vi "Simulated Car Client.vi"(7 "stop signal":refnum<user-event>, 10 "project namespace":string="LabVIEWDemo", 11 "Client Name":string="Car") -> ()   [LabVIEW 2017]
uses:
  Car/Car State -- enum.ctl
  TrafficMap/TrafficMap.lvclass/TrafficMap.ctl
  <vilib>/LabVIEW Open Source Project/MQTT Broker/Client/Client.lvclass
  C:/Program Files (x86)/National Instruments/LabVIEW 2017/vi.lib/LabVIEW Open Source Project/MQTT Broker/MQTT_Base/MQTT_Base.lvclass
  <vilib>/LabVIEW Open Source Project/MQTT Broker/Control Packets/PUBLISH/PUBLISH.lvclass
  C:/Program Files (x86)/National Instruments/LabVIEW 2017/vi.lib/LabVIEW Open Source Project/MQTT Broker/Control Packets/ControlPacket/ControlPacket.lvclass
  typedefs/Node Type -- enum.ctl
  TrafficMap/TrafficMap.lvclass
  typedefs/RequestPayload -- cluster.ctl
  typedefs/ResponsePayload -- cluster.ctl
  Serializer.JKI-JSON/Serializer.JKI-JSON.lvclass
  C:/Program Files (x86)/National Instruments/LabVIEW 2017/vi.lib/LabVIEW Open Source Project/Serializer/Serializer/Serializer.lvclass
  <vilib>/LabVIEW Open Source Project/MQTT Broker/MQTT_Base/MQTT_Base.lvclass/MQTT_Base.ctl
  <vilib>/LabVIEW Open Source Project/MQTT Broker/Client/Client.lvclass/Client.ctl
  <vilib>/LabVIEW Open Source Project/MQTT Broker/Control Packets/CONNECT/ConnectFlags -- cluster.ctl
  typedefs/ConnectPayload-- cluster.ctl
  typedefs/DisconnectPayload-- cluster.ctl
  <vilib>/LabVIEW Open Source Project/MQTT Broker/Control Packets/ControlPacket/ControlPacket.lvclass/ControlPacket.ctl
  0d705227-134d-4031-8d1e-e35da49b8ba8.vi
  580889ff-0a4c-41a4-b259-1db762517910.vi
  3d3687d4-2784-4a3f-94ff-e25152285f29.vi
  45bbbbd6-bbd6-4c9d-8aa1-54a553140d59.vi
  c7907ea9-6b4e-410e-be68-a96135e16753.vi
  a8e81dbf-d079-406f-abbd-3f6e0d275bc5.vi
  b830538a-2e83-4cc7-9605-dce1a29f0d38.vi
  <vilib>/LabVIEW Open Source Project/Serializer/Serializer.FlattenedString/Serializer.FlattenedString.lvclass
  <vilib>/LabVIEW Open Source Project/MQTT Broker/MQTT_Base/Decode Publish Package.vi
  <vilib>/LabVIEW Open Source Project/Serializer/Serializer/Serializer.lvclass
  <vilib>/LabVIEW Open Source Project/MQTT Broker/MQTT_Base/MQTT_Base.lvclass
  <vilib>/LabVIEW Open Source Project/MQTT Broker/Control Packets/ControlPacket/ControlPacket.lvclass
  <vilib>/LabVIEW Open Source Project/MQTT Broker/Control Packets/CONNECT/CONNECT.lvclass
  <vilib>/addons/_JKI.lib/Serialization/JSON/JKI JSON Serialization.lvlib
  Car/Car.lvclass
panel:
  out "Incoming topic":string
  out "Nb Cars in Current Zone":u32(knob) scale=0.0..10.0
  out "Zone registered":string
  in  "Map Update":bool
  out "Map":u16[][](graph)
  in  "Zones":u16(ring) items=["A", "B", "C", "D"]
  in  "Set Zone":bool
  in  "car state":T1
  in  "List Zones":bool
  out "Raw Packet String":string
  out "Payload":variant
  in  "Car Client Status":i32(listbox)
  out "Topic":string
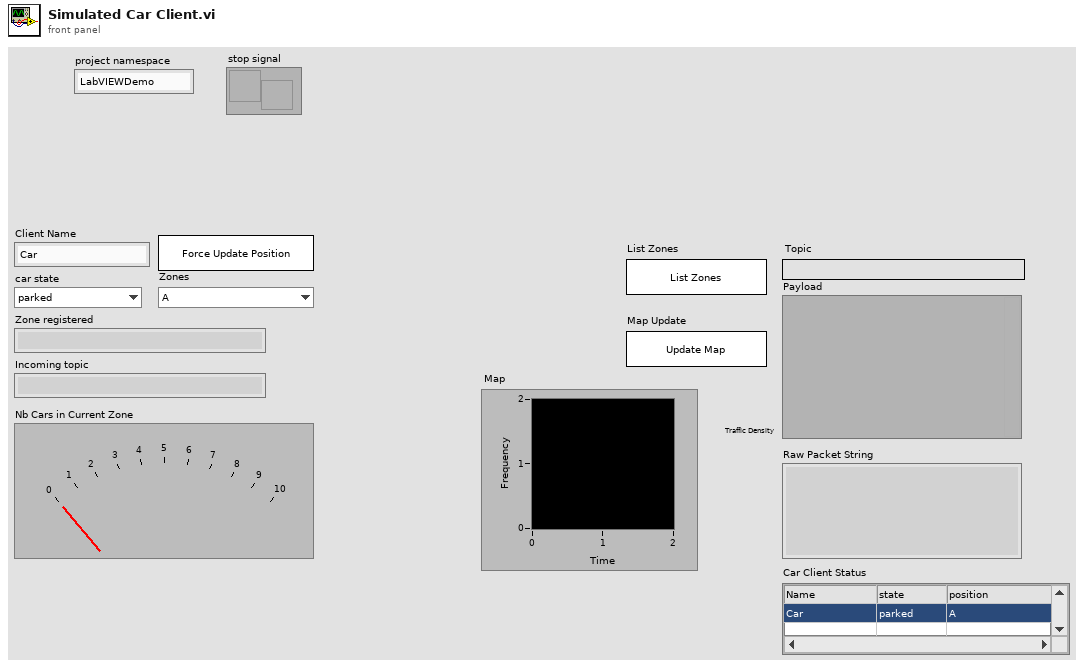
[diagram p1: front panel]
types:
  T1 = typedef "Car.lvclass/Car State -- enum.ctl" = enum16{"parked", "driving"}
  T2 = enum32{"Invalid", "Standard", "Closed", "Hidden", "Minimized", "Maximized"}
  T3 = enum32{"invalid app kind", "Development System", "Run Time System", "Student Edition", "Embedded LabVIEW", "Evaluation", "Custom"}
  T4 = typedef "ResponsePayload -- cluster.ctl" = cluster{"request":string, "reply":variant}
  T5 = typedef "CONNECT.lvclass/ConnectFlags -- cluster.ctl" = cluster{"Reserved":bool, "Clean Session":bool, "Will Flag":bool, "Will QoS 1":bool, "Will QoS 2":bool, "Will Retain":bool, "Password Flag":bool, "User Name Flag":bool}
  T6 = cluster{"Will Topic":string, "Will Message":string, "Username":string, "Password":string}
  T7 = typedef "RequestPayload -- cluster.ctl" = cluster{"request":string, "reply-to":string}
  T8 = typedef "ConnectPayload-- cluster.ctl" = cluster{"Node type":string}
  T9 = typedef "DisconnectPayload-- cluster.ctl" = cluster{"timestamp":string}
  T10 = typedef "Node Type -- enum.ctl" = enum16{"Car", "Hub", "Sensor", "Relay"}
  T11 = cluster{"Core":cluster{"Current VI Reference":refnum<vi>, "Close Panel on Exit?":bool}, "server address":string, "project namespace":string, "Client Name":string, "Node type":T10, "Client":refnum<class "Client.lvclass">, "Close on MQTT Disconnection?":bool, "Hub Name":string, "AppMessage":refnum<class "PUBLISH.lvclass">, "stop signal":refnum<user-event>, "TrafficMap":refnum<class "TrafficMap.lvclass">, "Request":T7}
  T12 = typedef "CONNACK.lvclass/Connect Return Code -- enum.ctl" = enum16{"Connection accepted", "Unacceptable protocol version", "Identifier Rejected", "Server Unavailable", "Bad Username or Password", "Not Authorized"}
  T13 = cluster{"Current VI Reference":refnum<vi>, "Close Panel on Exit?":bool}
  T14 = typedef "MQTT Server.lvlib/Client.lvclass/Public Events -- cluster.ctl" = cluster{"Connection Status":refnum<user-event>, "Connected":refnum<user-event>, "Application Message":refnum<user-event>}
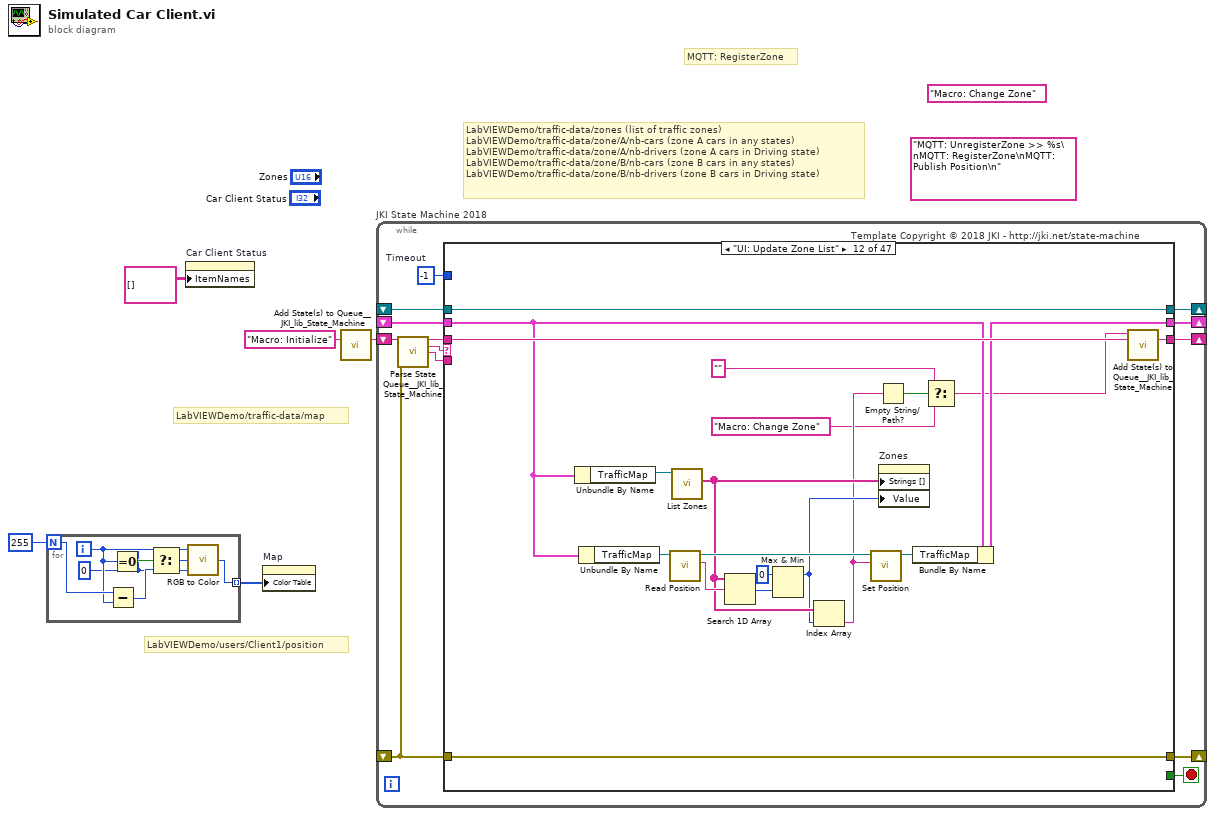
[diagram p0: block diagram]
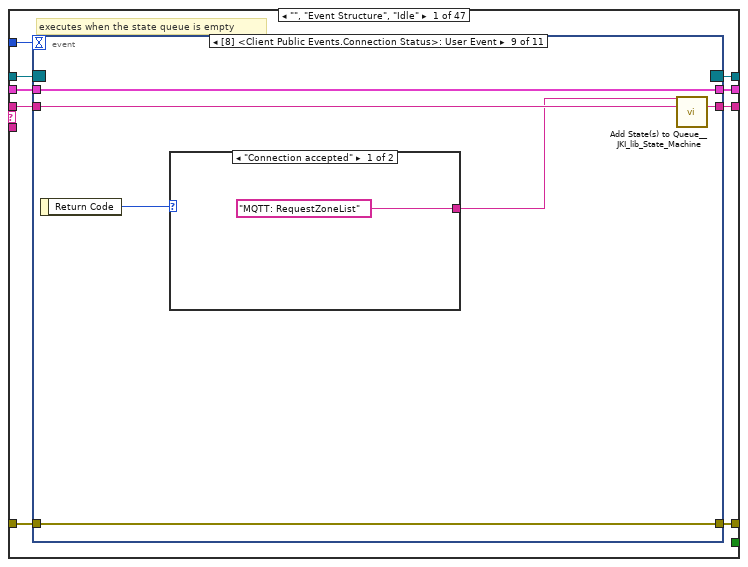
[diagram p2: hidden frame]
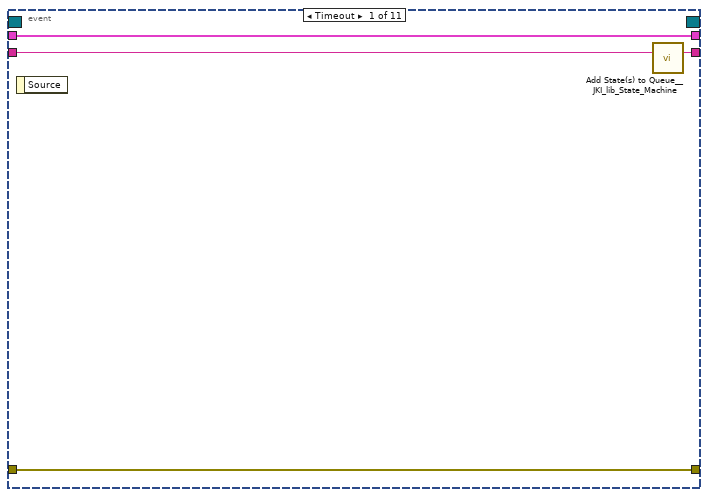
[diagram p3: hidden frame]
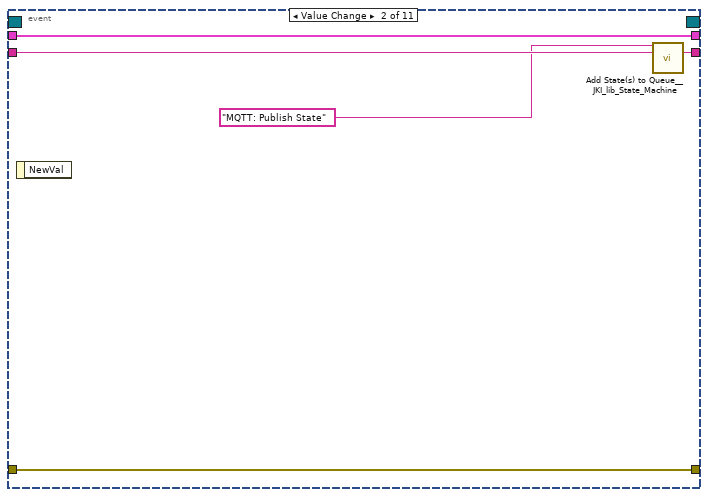
[diagram p4: hidden frame]
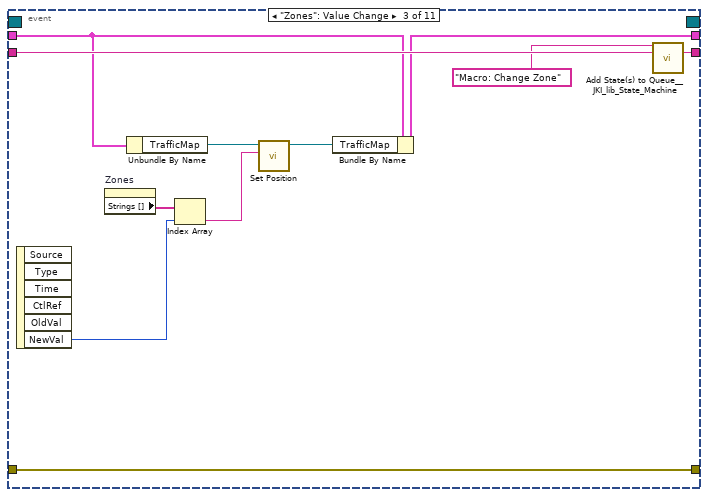
[diagram p5: hidden frame]
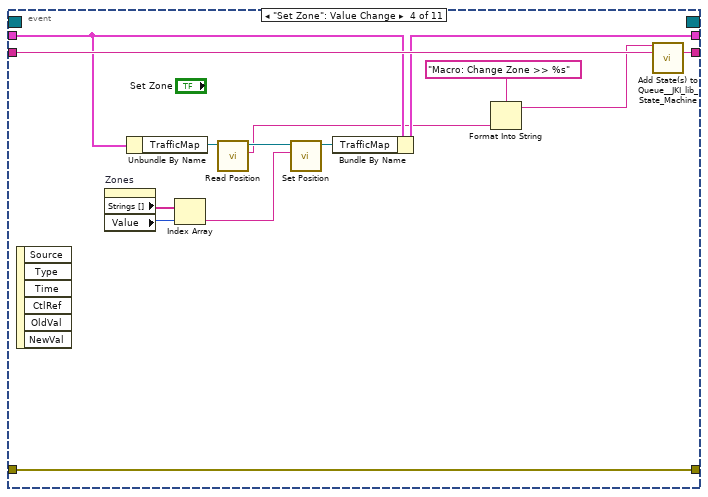
[diagram p6: hidden frame]
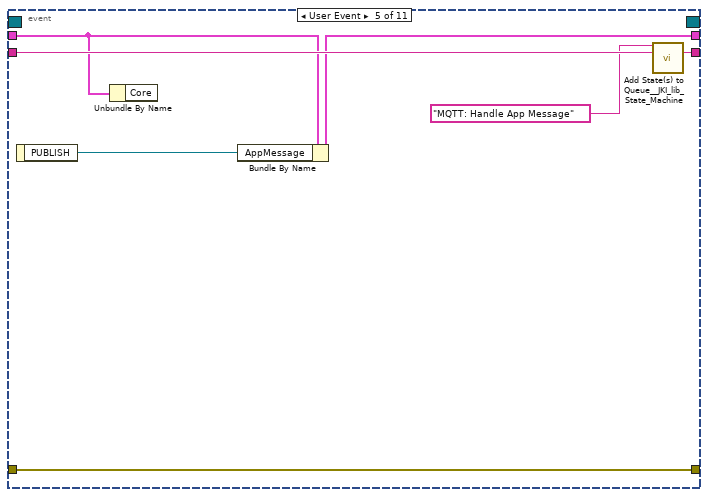
[diagram p7: hidden frame]
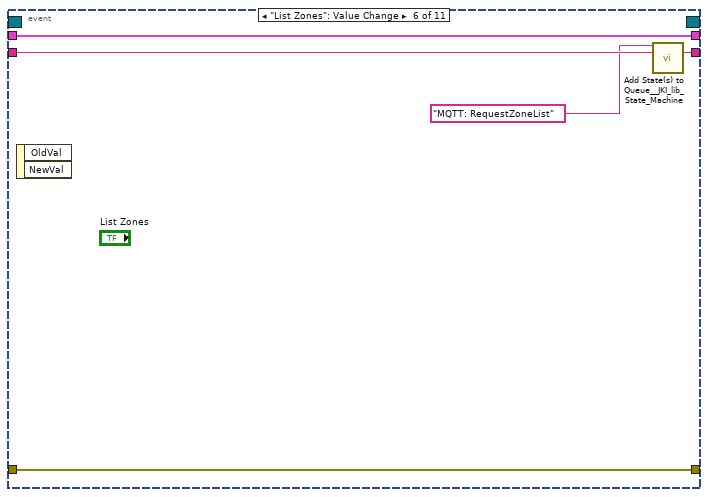
[diagram p8: hidden frame]
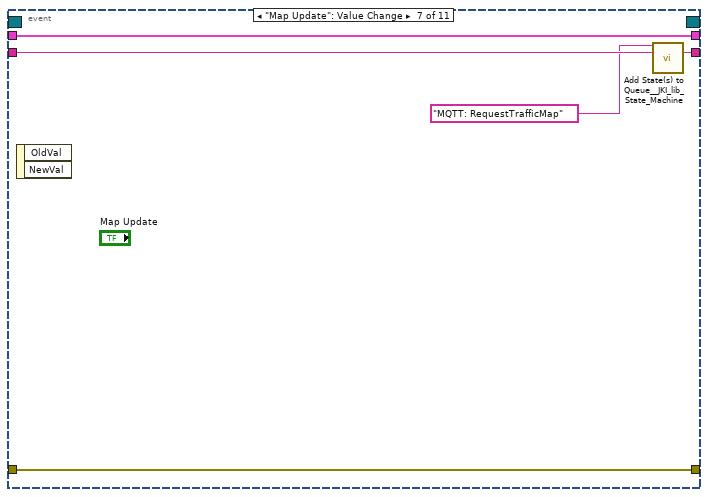
[diagram p9: hidden frame]
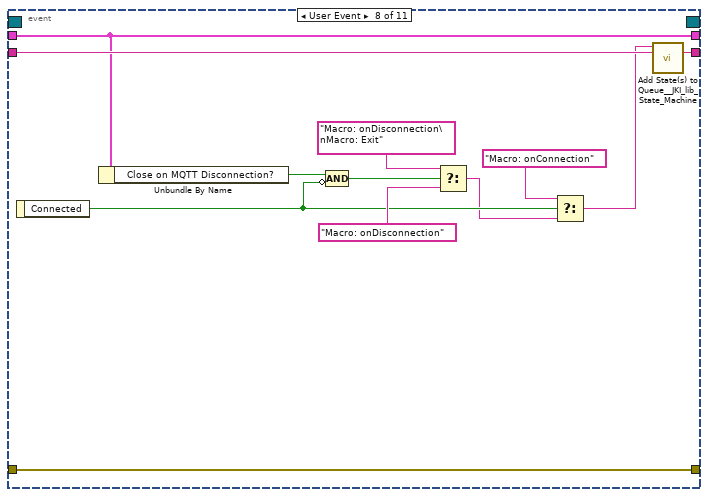
[diagram p10: hidden frame]
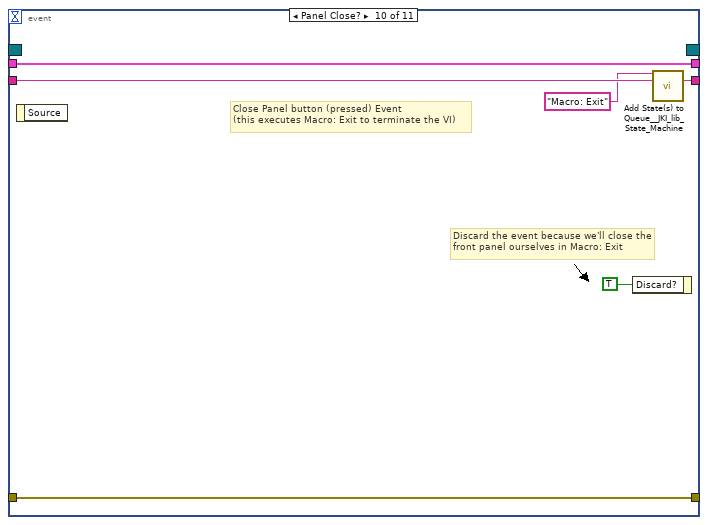
[diagram p12: hidden frame]
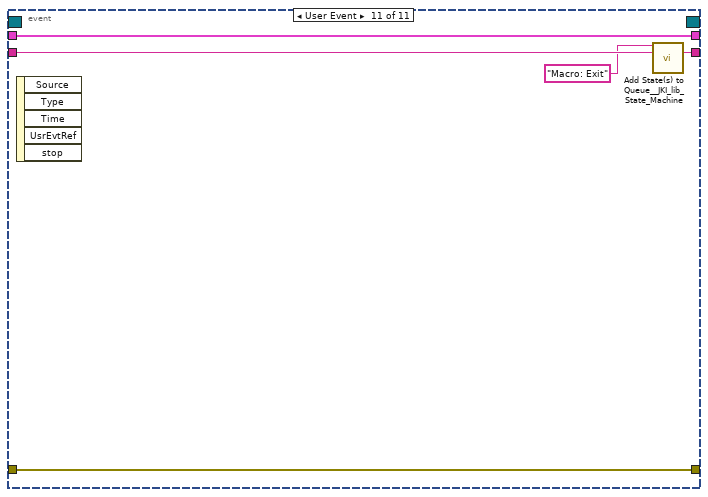
[diagram p13: hidden frame]
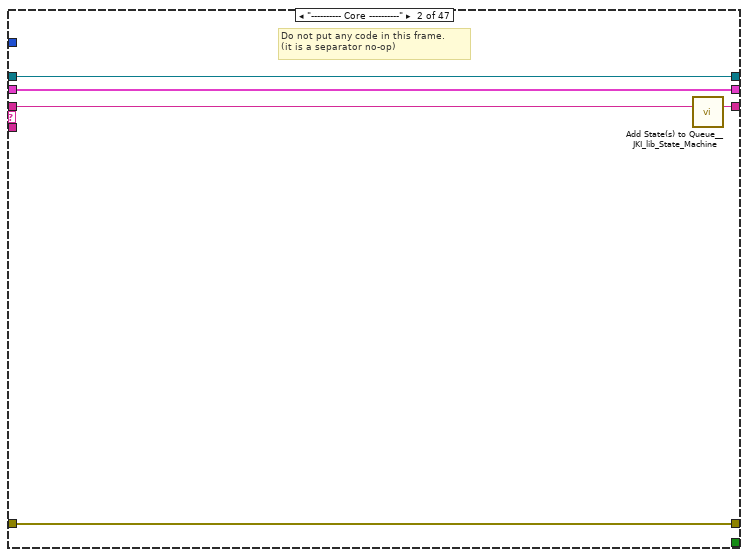
[diagram p14: hidden frame]
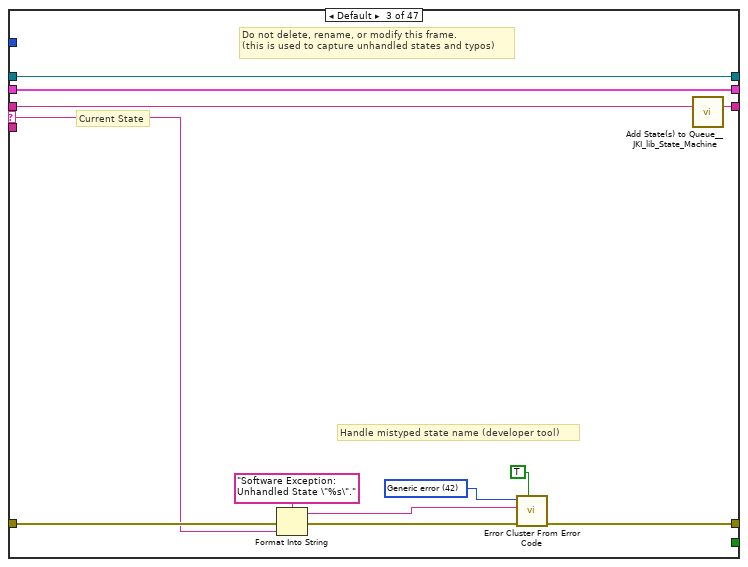
[diagram p15: hidden frame]
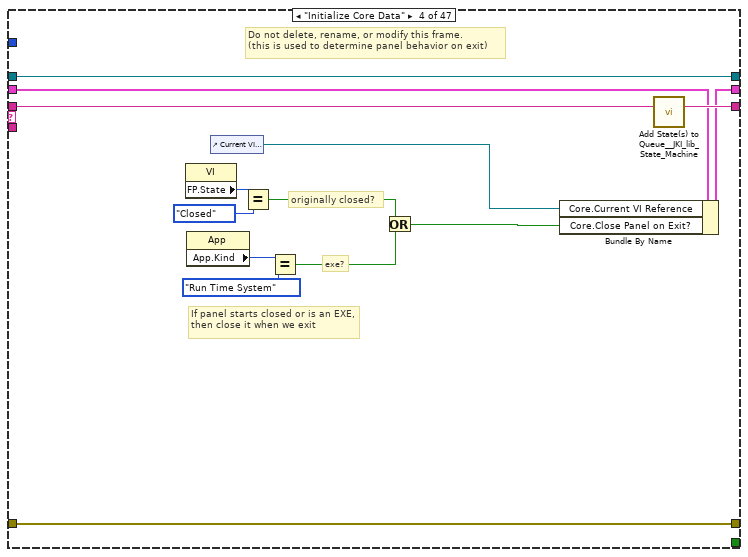
[diagram p16: hidden frame]
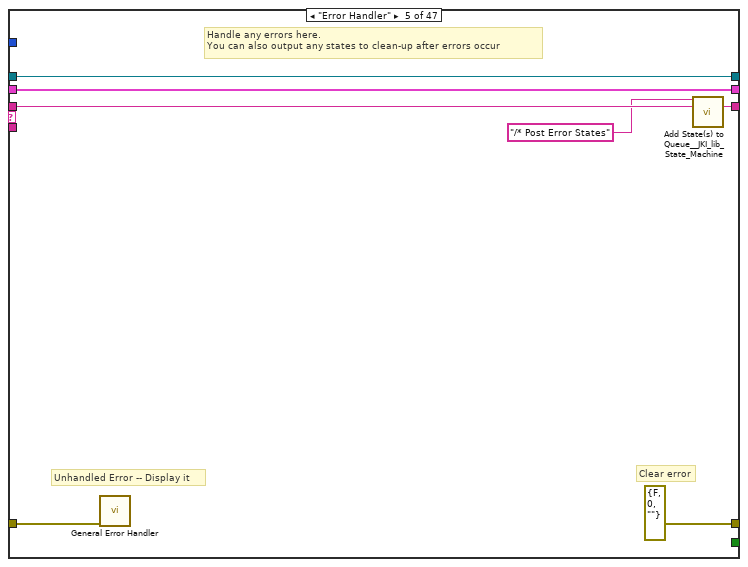
[diagram p17: hidden frame]
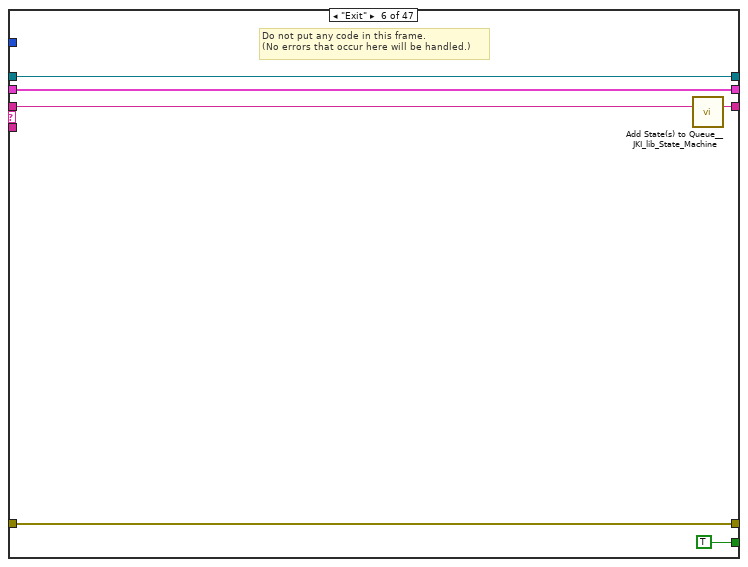
[diagram p18: hidden frame]
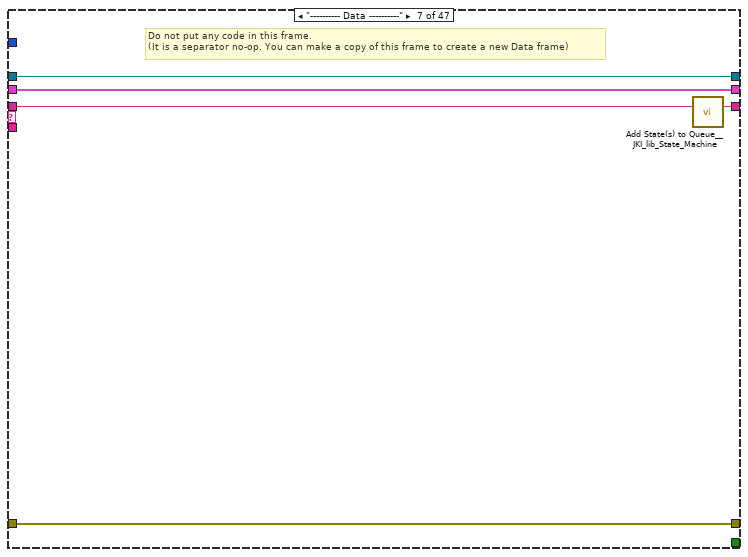
[diagram p19: hidden frame]
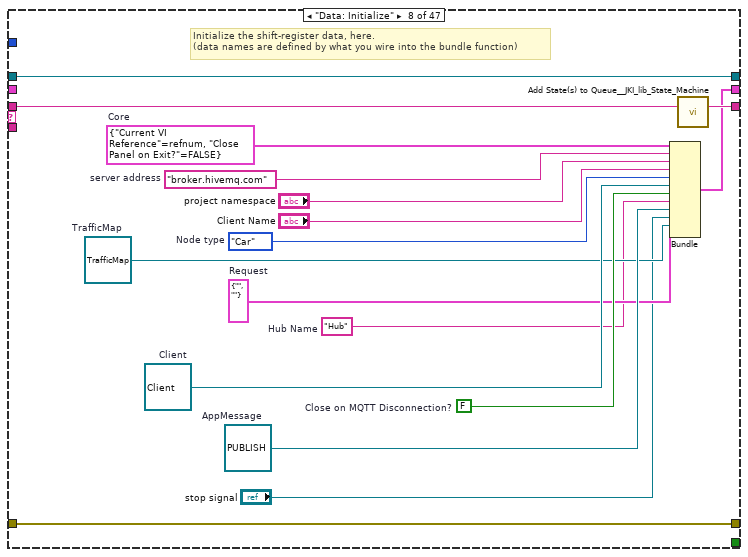
[diagram p20: hidden frame]
diagram:
  (unwired) "MQTT: UnregisterZone >> %s\nMQTT: RegisterZone\nMQTT: Publish Position\n"
  (unwired) "Macro: Change Zone"
  # "MQTT: RegisterZone"
  # "LabVIEWDemo/traffic-data/zones (list of traffic zones)\nLabVIEWDemo/traffic-data/zone/A/nb-cars (zone A cars in any states)\nLabVIEWDemo/traffic-data/zone/A/nb-drivers (zone A cars in Driving state)\nLabVIEWDemo/traffic-data/zone/B/nb-cars (zone B cars in any states)\nLabVIEWDemo/traffic-data/zone/B/nb-drivers (zone B cars in Driving state)"
  # "LabVIEWDemo/traffic-data/map"
  # "LabVIEWDemo/users/Client1/position"
  n1 = for {
    N: 255 -> [w11]
    tunnel: [w12] -> w1 mode=indexing
    i -> [w10]
    w7 = u8 0 ("B")
    n2 = Subtract(x=w11, y=w10) -> (x-y=w8:i32)
    n3 = Equal To 0?(x=w10) -> (x = 0?=w9:bool)
    n4 = Select(t=w7, s=w9, f=w8) -> (s? t:f=w6:i32)
    n5 = call <vilib>:"RGB to Color.vi"("B"=w7, "G"=w6, "R"=w10) -> ("Color"=w12:u32)
  }
  n6 = property on="Car Client Status" class="MCListbox (strict)"("ItemNames"=string[][] [] ("Item Names")) -> ()  [unwired: 2 in, 2 out]
  n7 = property on="Map" class="IntGraph (strict)"("Color Table"=w1) -> ()  [unwired: 2 in, 2 out]
  n8 = call <vilib>:"Add State(s) to Queue__JKI_lib_State_Machine.vi"("State(s) in (\"\")"="Macro: Initialize") -> ("States Out"=w4:string)  [unwired: 14 in]
  n9 = while "JKI State Machine 2018" {
    shift-right: [w18] -> _
    shift-left: _ -> [w17]
    shift-right: [w21] -> _
    shift-left: _ -> [w15]
    shift-right: [w20] -> _
    shift-left: w4 -> [w22]
    shift-right: [w14] -> _
    shift-left: _ -> [w13]
    stop <- w19 stop-if-true
    w16 = -1  # Timeout
    # "Template Copyright © 2018 JKI - http://jki.net/state-machine"
    n10 = call <vilib>:"Parse State Queue__JKI_lib_State_Machine.vi"("State Queue"=w22, "Error In (no error)"=w15) -> ("Remaining States"=w24:string, "Current State"=w25:string, "Arguments"=w23:string)  [unwired: 11 in]
    n11 = case shown="\"UI: Update Zone List\"" w25 {
      selector: w25 -> [_ _ w122 _ _ _ _ _ _ _ _ _ _ _ _ _ _ _ _ _ _ _ _ _ _ _ _ _ _ _ _ _ _ _ _ _ _ _ _ _ _ _ _ _ _ _ _]
      tunnel: w24 -> [w34 w120 w126 w146 w153 w159 w164 w181 w189 w194 w202 w222 w229 w236 w248 w318 w324 w330 w336 w344 w349 w355 w367 w372 w380 w386 w393 w398 w413 w434 w445 w457 w481 w494 w507 w519 w545 w560 w575 w593 w611 w628 w644 w665 w830 w836 w843]
      tunnel: w23 -> [_ _ _ _ _ _ _ _ _ _ _ _ _ w231 w242 _ _ _ _ w337 _ _ _ _ _ _ _ _ _ _ _ _ _ _ _ w509 _ _ _ _ _ _ _ _ _ _ _]
      tunnel: w17 -> [w32 w117 w124 w139 w150 w157 w161 _ w184 w191 w200 w209 w225 w234 w244 w315 w321 w327 w333 w341 w346 w352 w364 w369 w374 w382 w389 w395 w400 w431 w443 w454 w478 w491 w504 w510 w538 w557 w572 w590 w608 w625 w641 w651 w827 w831 w841]
      tunnel: [w31 w118 w128 w143 errorcluster {"status"=FALSE, "code"=0, "source"=""} ("error out") w156 w162 w178 w185 w192 w199 w220 w227 w232 w245 w316 w322 w328 w334 w342 w347 w353 w365 w370 w378 w384 w391 w396 w404 w432 w435 w447 w472 w483 w499 w512 w534 w548 w563 w583 w601 w616 w632 w662 w822 w832 w838] -> w21
      tunnel: w15 -> [w30 w118 w127 w143 w149 w156 w162 w178 w186 w192 w199 w220 w227 w233 w246 w316 w322 w328 w334 w342 w347 w353 w365 w370 w378 w384 w391 w396 w405 w432 w441 w450 w473 w484 w500 w513 w535 w549 w564 w584 w602 w617 w633 w662 w820 w833 w839]
      tunnel: [w33 w119 w125 w145 w152 w158 w163 w180 w188 w193 w201 w221 w228 w235 w247 w317 w323 w329 w335 w343 w348 w354 w366 w371 w379 w385 w392 w397 w412 w433 w444 w456 w480 w493 w506 w518 w544 w559 w574 w592 w610 w627 w643 w664 w829 w835 w842] -> w20
      tunnel: [_ _ _ _ _ TRUE _ _ _ _ _ _ _ _ _ _ _ _ _ _ _ _ _ _ _ _ _ _ _ _ _ _ _ _ _ _ _ _ _ _ _ _ _ _ _ _ _] -> w19
      tunnel: [w29 w117 w124 w144 w150 w157 w161 w179 w184 w191 w200 w208 w225 w234 w244 w315 w321 w327 w333 w341 w346 w352 w364 w369 w373 w382 w389 w395 w411 w431 w442 w455 w479 w492 w505 w517 w543 w558 w573 w591 w609 w626 w642 w650 w828 w831 w841] -> w18
      tunnel: w16 -> [w28 _ _ _ _ _ _ _ _ _ _ _ _ _ _ _ _ _ _ _ _ _ _ _ _ _ _ _ _ _ _ _ _ _ _ _ _ _ _ _ _ _ _ _ _ _ _]
      tunnel: w13 -> [w27 w116 w121 w133 w147 w154 w160 w173 w183 w190 w198 w219 w226 w230 w241 w314 w319 w325 w331 w340 w345 w350 w356 w368 w377 w383 w390 w394 w410 w430 w440 _ w477 w490 w503 w516 w542 w556 w571 w589 w607 w624 w640 w663 w826 w834 w837]
      tunnel: [w26 w116 w121 w133 w147 w154 w160 w173 w183 w190 w198 w219 w226 w230 w241 w314 w319 w325 w331 w340 w345 w350 w356 w368 w377 w383 w390 w394 w410 w430 w440 w449 w477 w490 w503 w516 w542 w556 w571 w589 w607 w624 w640 w663 w826 w834 w837] -> w14
      frame "", "Event Structure", "Idle" {
        # "executes when the state queue is empty"
        n12 = event shown="[8] <Client Public Events.Connection Status>: User Event" {
          selector: w27 -> [_ _ _ _ _ _ _ _ _ _ _]
          dyn-events: [_ _ _ _ _ _ _ _ _ _ _] -> w26
          timeout: w28 -> [_ _ _ _ _ _ _ _ _ _ _]
          tunnel: w34 -> [w38 w43 w54 w68 w75 w80 w85 w97 w103 w110 w115]
          tunnel: [w37 w42 w53 w67 w74 w79 w84 w96 w102 w109 w114] -> w33
          tunnel: w32 -> [w35 w40 w50 w65 w71 w76 w81 w94 w100 w107 w112]
          tunnel: [w36 w41 w52 w66 w73 w78 w83 w95 w101 w108 w113] -> w31
          tunnel: w30 -> [w36 w41 w52 w66 w73 w78 w83 w95 w101 w108 w113]
          tunnel: [w35 w40 w49 w64 w70 w76 w81 w94 w100 w107 w112] -> w29
          event Timeout {
            n13 = event-data() -> ()  [unwired: 1 in, 1 out]
            n14 = call <vilib>:"Add State(s) to Queue__JKI_lib_State_Machine.vi"("State(s) in (\"\")"=w38) -> ("States Out"=w37:string)  [unwired: 14 in]
          }
          event Value Change {
            n15 = event-data() -> ()  [unwired: 1 in, 1 out]
            n16 = call <vilib>:"Add State(s) to Queue__JKI_lib_State_Machine.vi"("State(s) in Front (\"\")"="MQTT: Publish State", "State(s) in (\"\")"=w43) -> ("States Out"=w42:string)  [unwired: 13 in]
          }
          event "Zones": Value Change {
            n17 = event-data() -> ("NewVal"=w44:u16)  [unwired: 1 in, 5 out]
            n18 = property on="Zones" class="Ring (strict)"() -> ("Strings []"=w46:string[])  [unwired: 2 in, 2 out]
            n19 = Unbundle By Name(w50) -> ("TrafficMap"=w48:refnum<class "TrafficMap.lvclass">)
            n20 = Index Array(array=w46, index=w44) -> (element=w45:string)
            n21 = call "Set Position.vi"("Position"=w45, "TrafficMap in"=w48) -> ("TrafficMap out"=w47:refnum<class "TrafficMap.lvclass">)  [unwired: 8 in, 1 out]
            n22 = Bundle By Name(cluster=w50, "TrafficMap"=w47) -> (w49:T11)
            n23 = call <vilib>:"Add State(s) to Queue__JKI_lib_State_Machine.vi"("State(s) in Front (\"\")"="Macro: Change Zone", "State(s) in (\"\")"=w54) -> ("States Out"=w53:string)  [unwired: 13 in]
          }
          event "Set Zone": Value Change {
            n24 = event-data() -> ()  [unwired: 1 in, 6 out]
            n25 = property on="Zones" class="Ring (strict)"() -> ("Strings []"=w62:string[], "Value"=w60:u16)  [unwired: 2 in, 2 out]
            n26 = Unbundle By Name(w65) -> ("TrafficMap"=w59:refnum<class "TrafficMap.lvclass">)
            n27 = Index Array(array=w62, index=w60) -> (element=w61:string)
            n28 = call "Read Position.vi"("TrafficMap in"=w59) -> ("Position"=w57:string, "TrafficMap out"=w58:refnum<class "TrafficMap.lvclass">)  [unwired: 8 in, 1 out]
            n29 = call "Set Position.vi"("Position"=w61, "TrafficMap in"=w58) -> ("TrafficMap out"=w63:refnum<class "TrafficMap.lvclass">)  [unwired: 8 in, 1 out]
            n30 = Bundle By Name(cluster=w65, "TrafficMap"=w63) -> (w64:T11)
            n31 = Format Into String(format string="Macro: Change Zone >> %s", w57) -> (resulting string=w55:string)  [unwired: 2 in, 1 out]
            n32 = call <vilib>:"Add State(s) to Queue__JKI_lib_State_Machine.vi"("State(s) in Front (\"\")"=w55, "State(s) in (\"\")"=w68) -> ("States Out"=w67:string)  [unwired: 13 in]
          }
          event User Event {
            n33 = event-data() -> ("PUBLISH"=w72:refnum<class "PUBLISH.lvclass">)  [unwired: 1 in]
            n34 = Unbundle By Name(w71) -> ()  [unwired: 1 out]
            n35 = Bundle By Name(cluster=w71, "AppMessage"=w72) -> (w70:T11)
            n36 = call <vilib>:"Add State(s) to Queue__JKI_lib_State_Machine.vi"("State(s) in Front (\"\")"="MQTT: Handle App Message", "State(s) in (\"\")"=w75) -> ("States Out"=w74:string)  [unwired: 13 in]
          }
          event "List Zones": Value Change {
            n37 = event-data() -> ()  [unwired: 1 in, 2 out]
            n38 = call <vilib>:"Add State(s) to Queue__JKI_lib_State_Machine.vi"("State(s) in Front (\"\")"="MQTT: RequestZoneList", "State(s) in (\"\")"=w80) -> ("States Out"=w79:string)  [unwired: 13 in]
          }
          event "Map Update": Value Change {
            n39 = event-data() -> ()  [unwired: 1 in, 2 out]
            n40 = call <vilib>:"Add State(s) to Queue__JKI_lib_State_Machine.vi"("State(s) in Front (\"\")"="MQTT: RequestTrafficMap", "State(s) in (\"\")"=w85) -> ("States Out"=w84:string)  [unwired: 13 in]
          }
          event User Event {
            n41 = event-data() -> ("Connected"=w89:bool)  [unwired: 1 in]
            n42 = Unbundle By Name(w94) -> ("Close on MQTT Disconnection?"=w93:bool)
            n43 = Compound Arithmetic op=AND(w93, invert w89) -> (w92:bool)
            n44 = Select(t="Macro: onDisconnection\nMacro: Exit", s=w92, f="Macro: onDisconnection" ("t")) -> (s? t:f=w87:string)
            n45 = Select(t="Macro: onConnection", s=w89, f=w87) -> (s? t:f=w86:string)
            n46 = call <vilib>:"Add State(s) to Queue__JKI_lib_State_Machine.vi"("State(s) in Front (\"\")"=w86, "State(s) in (\"\")"=w97) -> ("States Out"=w96:string)  [unwired: 13 in]
          }
          event User Event {
            n47 = event-data() -> ("Return Code"=w99:T12)  [unwired: 1 in]
            n48 = case shown="\"Connection accepted\"" w99 {
              tunnel: ["MQTT: RequestZoneList" ("format string") _] -> w98
              frame "Connection accepted" {
              }
              frame Default {
              }
            }
            n49 = call <vilib>:"Add State(s) to Queue__JKI_lib_State_Machine.vi"("State(s) in Front (\"\")"=w98, "State(s) in (\"\")"=w103) -> ("States Out"=w102:string)  [unwired: 13 in]
          }
          event Panel Close? {
            # "Discard the event because we'll close the front panel ourselves in Macro: Exit"
            # "Close Panel button (pressed) Event\n(this executes Macro: Exit to terminate the VI)"
            n50 = event-data() -> ()  [unwired: 1 in, 1 out]
            n51 = event-data("Discard?"=TRUE) -> ()  [unwired: 1 in, 1 out]
            n52 = call <vilib>:"Add State(s) to Queue__JKI_lib_State_Machine.vi"("State(s) in Front (\"\")"="Macro: Exit", "State(s) in (\"\")"=w110) -> ("States Out"=w109:string)  [unwired: 13 in]
          }
          event User Event {
            n53 = event-data() -> ()  [unwired: 1 in, 5 out]
            n54 = call <vilib>:"Add State(s) to Queue__JKI_lib_State_Machine.vi"("State(s) in Front (\"\")"="Macro: Exit", "State(s) in (\"\")"=w115) -> ("States Out"=w114:string)  [unwired: 13 in]
          }
        }
      }
      frame "---------- Core ----------" {
        # "Do not put any code in this frame.\n(it is a separator no-op)"
        n55 = call <vilib>:"Add State(s) to Queue__JKI_lib_State_Machine.vi"("State(s) in (\"\")"=w120) -> ("States Out"=w119:string)  [unwired: 14 in]
      }
      frame Default {
        w131 = 42 items=["No error", "Argument error", "Memory is full", "Out of zone", "End of file", "File already open", "Generic file I/O error", "File not found", "File permission error", "Disk is full", "Duplicate path", "Too many files open", "System feature not enabled", "Resource file not found", "Cannot add resource", "Resource not found", "Image not found", "Image memory error", "Pen does not exist", "Config type invalid", "Config token not found", "Config parse error", "Config memory error", "Bad external code format", "Bad external code offset", "External code not present", "Null window", "Destroy window error", "Null menu", "Print aborted", "Bad print record", "Print driver error", "Windows error during printing", "Memory error during printing", "Print dialog error", "Generic print error", "Invalid device refnum", "Device not found", "Device parameter error", "Device unit error", "Cannot open device", "Device call aborted", "Generic error", "Cancelled by user", "Object ID too low", "Object ID too high", "Object not in heap", "Unknown heap", "Unknown object (invalid DefProc)", "Unknown object (DefProc not in table)", "Message out of range", "Invalid (null) method", "Unknown message", "Manager call not supported", "Bad address", "Network operation in progress", "Network operation timed out", "Connection is busy", "Network attribute not supported", "Network error", "Address in use", "System out of memory", "Connection aborted", "Connection refused", "Not connected", "Already connected", "Connection closed", "Initialization error (interapplication manager)", "Bad occurrence", "Wait on unbound occurrence handler", "Occurrence queue overflow", "Datalog type conflict", "Unused", "Unrecognized type (interapplication manager)", "Memory corrupt", "Failed to make temporary DLL", "Old CIN version", "Drag socket not found", "Failed to load drop-object", "Failed to register OLE object", "Failed to release OLE object", "Format specifier type mismatch", "Unknown format specifier", "Too few format specifiers", "Too many format specifiers", "Scan failed", "Newer CIN version", "Error converting to variant", "Runtime menu error", "Password tampered", "Variant attribute not found", "Incompatible variant data type", "Event data is not available", "Event Store is not present", "Occurrence is not found", "Event Queue is not created", "Event info is not available", "Refnum passed is NULL", "Error retrieving Class GUID", "Error retrieving CoClass GUID", "Error retrieving TypeLib GUID.", "Bad built application magic bytes.", "Specific driver is different from the specific driver associated with the Logical Name.", "There is no session opened to the class driver.", "Max Error", "MAX - Error with config objects", "MAX - Error loading configuration", "MAX - Group not supported"]
        # "Current State"
        # "Do not delete, rename, or modify this frame.\n(this is used to capture unhandled states and typos)"
        # "Handle mistyped state name (developer tool)"
        n56 = Format Into String(format string="Software Exception: Unhandled State \"%s\"." ("message"), error in=w127, w122) -> (resulting string=w130:string, error out=w129:errorcluster)  [unwired: 1 in]
        n57 = call <vilib>:"Error Cluster From Error Code.vi"("show call chain? (False)"=TRUE, "error in (no error)"=w129, "error message (\"\")"=w130, "error code (0)"=w131) -> ("error out"=w128:errorcluster)  [unwired: 5 in]
        n58 = call <vilib>:"Add State(s) to Queue__JKI_lib_State_Machine.vi"("State(s) in (\"\")"=w126) -> ("States Out"=w125:string)  [unwired: 14 in]
      }
      frame "Initialize Core Data" {
        # "Do not delete, rename, or modify this frame.\n(this is used to determine panel behavior on exit)"
        # "originally closed?"
        # "exe?"
        # "If panel starts closed or is an EXE, then close it when we exit"
        n59 = property class="VI"() -> ("FP.State"=w136:T2)  [unwired: 2 in, 2 out]
        n60 = property class="App"() -> ("App.Kind"=w142:T3)  [unwired: 2 in, 2 out]
        n61 = control-ref of="Current VI Reference"() -> (w137:refnum<vi>)
        n62 = Equal?(x=w136, y=T2."Closed" ("Front Panel Window:State")) -> (x = y?=w134:bool)
        n63 = Equal?(x=w142, y=T3."Run Time System" ("Application:Kind")) -> (x = y?=w140:bool)
        n64 = Or(x=w134, y=w140) -> (x .or. y?=w138:bool)
        n65 = Bundle By Name(cluster=w139, "Core.Current VI Reference"=w137, "Core.Close Panel on Exit?"=w138) -> (w144:T11)
        n66 = call <vilib>:"Add State(s) to Queue__JKI_lib_State_Machine.vi"("State(s) in (\"\")"=w146) -> ("States Out"=w145:string)  [unwired: 14 in]
      }
      frame "Error Handler" {
        # "Unhandled Error -- Display it"
        # "Handle any errors here.\nYou can also output any states to clean-up after errors occur"
        # "Clear error"
        n67 = call <vilib>:"General Error Handler.vi"("error in (no error)"=w149) -> ()  [unwired: 10 in, 5 out]
        n68 = call <vilib>:"Add State(s) to Queue__JKI_lib_State_Machine.vi"("State(s) in Front (\"\")"="/* Post Error States", "State(s) in (\"\")"=w153) -> ("States Out"=w152:string)  [unwired: 13 in]
      }
      frame "Exit" {
        # "Do not put any code in this frame.\n(No errors that occur here will be handled.)"
        n69 = call <vilib>:"Add State(s) to Queue__JKI_lib_State_Machine.vi"("State(s) in (\"\")"=w159) -> ("States Out"=w158:string)  [unwired: 14 in]
      }
      frame "---------- Data ----------" {
        # "Do not put any code in this frame.\n(It is a separator no-op. You can make a copy of this frame to create a new Data frame)"
        n70 = call <vilib>:"Add State(s) to Queue__JKI_lib_State_Machine.vi"("State(s) in (\"\")"=w164) -> ("States Out"=w163:string)  [unwired: 14 in]
      }
      frame "Data: Initialize" {
        w167 = "Hub"  # Hub Name
        w168 = T7 {"request"="", "reply-to"=""}  # Request
        w169 = refnum<class "TrafficMap.lvclass"> refnum  # TrafficMap
        w170 = Node_Type_--_enum."Car"  # Node type
        w171 = refnum<class "PUBLISH.lvclass"> refnum  # AppMessage
        w172 = FALSE  # Close on MQTT Disconnection?
        w174 = refnum<class "Client.lvclass"> refnum  # Client
        w175 = "broker.hivemq.com"  # server address
        w176 = T13 {"Current VI Reference"=refnum, "Close Panel on Exit?"=FALSE}  # Core
        # "Initialize the shift-register data, here.\n(data names are defined by what you wire into the bundle function)"
        n71 = Bundle("Core"=w176, "server address"=w175, "project namespace"="project namespace", "Client Name"="Client Name", "Node type"=w170, "Client"=w174, "Close on MQTT Disconnection?"=w172, "Hub Name"=w167, "AppMessage"=w171, "stop signal"="stop signal", "TrafficMap"=w169, "Request"=w168) -> (w179:T11)  [unwired: 1 in]
        n72 = call <vilib>:"Add State(s) to Queue__JKI_lib_State_Machine.vi"("State(s) in (\"\")"=w181) -> ("States Out"=w180:string)  [unwired: 14 in]
      }
      frame "Data: Cleanup" {
        # "Cleanup any data and references, here.\n(this is called automatically, by the Macro: Exit)"
        n73 = Unbundle By Name(w184) -> ("Core.Current VI Reference"=w187:refnum<vi>)
        n74 = Close Reference(reference=w187, error in (no error)=w186) -> (error out=w185:errorcluster)
        n75 = call <vilib>:"Add State(s) to Queue__JKI_lib_State_Machine.vi"("State(s) in Front (\"\")"="//Sim: Destroy Stop Event", "State(s) in (\"\")"=w189) -> ("States Out"=w188:string)  [unwired: 13 in]
      }
      frame "---------- UI ----------" {
        # "Do not put any code in this frame.\n(It is a separator no-op. You can make a copy of this frame to create a new UI frame)"
        n76 = call <vilib>:"Add State(s) to Queue__JKI_lib_State_Machine.vi"("State(s) in (\"\")"=w194) -> ("States Out"=w193:string)  [unwired: 14 in]
      }
      frame "UI: Initialize" {
        w196 = u16 0 items=[""] ("Zones")
        # "Initialize the User Interface, here.\n(this is called automatically, by the Macro: Init)"
        n77 = local write "car state"(Car_State_--_enum."parked" ("car state")) -> ()
        n78 = property on="Zones" class="Ring (strict)"("Value"=w196, "Strings []"=string[] [] ("Zones")) -> ()  [unwired: 2 in, 2 out]
        n79 = call <vilib>:"Add State(s) to Queue__JKI_lib_State_Machine.vi"("State(s) in (\"\")"=w202) -> ("States Out"=w201:string)  [unwired: 14 in]
      }
      frame "UI: Update Zone List" {
        n80 = Unbundle By Name(w209) -> ("TrafficMap"=w218:refnum<class "TrafficMap.lvclass">)
        n81 = Unbundle By Name(w209) -> ("TrafficMap"=w214:refnum<class "TrafficMap.lvclass">)
        n82 = call "Read Position.vi"("TrafficMap in"=w214) -> ("Position"=w216:string, "TrafficMap out"=w215:refnum<class "TrafficMap.lvclass">)  [unwired: 8 in, 1 out]
        n83 = call "List Zones.vi"("TrafficMap in"=w218) -> ("Zones"=w211:string[])  [unwired: 7 in, 3 out]
        n84 = Search 1D Array(1D array=w211, element=w216) -> (index of element=w217:i32)  [unwired: 1 in]
        n85 = Max & Min(x=0, y=w217) -> (max(x,y)=w210:i32)  [unwired: 1 out]
        n86 = Index Array(array=w211, index=w210) -> (element=w207:string)
        n87 = call "Set Position.vi"("Position"=w207, "TrafficMap in"=w215) -> ("TrafficMap out"=w213:refnum<class "TrafficMap.lvclass">)  [unwired: 8 in, 1 out]
        n88 = Empty String/Path?(string/path=w207) -> (empty?=w206:bool)
        n89 = property on="Zones" class="Ring (strict)"("Strings []"=w211, "Value"=w210) -> ()  [unwired: 2 in, 2 out]
        n90 = Bundle By Name(cluster=w209, "TrafficMap"=w213) -> (w208:T11)
        n91 = Select(t="", s=w206, f="Macro: Change Zone") -> (s? t:f=w203:string)
        n92 = call <vilib>:"Add State(s) to Queue__JKI_lib_State_Machine.vi"("State(s) in Front (\"\")"=w203, "State(s) in (\"\")"=w222) -> ("States Out"=w221:string)  [unwired: 13 in]
      }
      frame "UI: Update Zone Map" {
        n93 = Unbundle By Name(w225) -> ("TrafficMap"=w224:refnum<class "TrafficMap.lvclass">)
        n94 = call "Read Map.vi"("TrafficMap in"=w224) -> ("Map"=→"Map":u16[][])  [unwired: 8 in, 2 out]
        n95 = call <vilib>:"Add State(s) to Queue__JKI_lib_State_Machine.vi"("State(s) in (\"\")"=w229) -> ("States Out"=w228:string)  [unwired: 14 in]
      }
      frame "UI: Cursor Set" {
        # "Argument"
        # "Set and Unset Cursor Busy.\n(Usage: \"UI: Cursor Set >> Busy|Idle\")"
        n96 = case shown="\"Idle\", Default" w231 {
          tunnel: w233 -> [w238 w240]
          tunnel: [w237 w239] -> w232
          frame "Idle", Default {
            n97 = call <vilib>:"Unset Busy.vi"("error in (no error)"=w238) -> ("error out"=w237:errorcluster)  [unwired: 10 in]
          }
          frame "Busy" {
            n98 = call <vilib>:"Set Busy.vi"("error in (no error)"=w240) -> ("error out"=w239:errorcluster)  [unwired: 9 in, 1 out]
          }
        }
        n99 = call <vilib>:"Add State(s) to Queue__JKI_lib_State_Machine.vi"("State(s) in (\"\")"=w236) -> ("States Out"=w235:string)  [unwired: 14 in]
      }
      frame "UI: Front Panel State" {
        # "Argument"
        # "Set Front Panel Open or Closed\n(Usage: \"UI: Front Panel State >> Open|Close\")"
        n100 = Unbundle By Name(w244) -> ("Core.Current VI Reference"=w243:refnum<vi>)
        n101 = case shown="\"Minimize\", \"Minimized\"" w242 {
          tunnel: w246 -> [w254 w269 w280 w293 w306]
          tunnel: [w256 w270 w282 w295 w308] -> w245
          tunnel: w243 -> [w255 w267 w281 w294 w307]
          frame "Open", "Standard", Default {
            w249 = T2."Standard" ("State")
            n102 = property class="VI"(reference=w255, error in=w254) -> (reference out=w252:refnum<vi>, error out=w253:errorcluster, "FP.State"=w251:T2)
            n103 = Not Equal?(x=w251, y=w249) -> (x != y?=w250:bool)
            n104 = case shown="True" w250 {
              tunnel: [w260 w262] -> w256
              tunnel: w253 -> [w259 w262]
              tunnel: w252 -> [w258 _]
              tunnel: w249 -> [w257 _]
              frame True {
                n105 = invoke class="VI" method="FP.Open"(reference=w258, error in=w259, "Activate"=TRUE, "State"=w257) -> (error out=w260:errorcluster)  [unwired: 1 in, 4 out]
              }
              frame False {
              }
            }
          }
          frame "Close", "Closed" {
            n106 = property class="VI"(reference=w267, error in=w269) -> (reference out=w266:refnum<vi>, error out=w268:errorcluster, "FP.State"=w264:T2)
            n107 = Not Equal?(x=w264, y=T2."Closed" ("Front Panel Window:State")) -> (x != y?=w263:bool)
            n108 = case shown="True" w263 {
              tunnel: [w271 w274] -> w270
              tunnel: w268 -> [w271 w273]
              tunnel: w266 -> [_ w272]
              frame False {
              }
              frame True {
                n109 = invoke class="VI" method="FP.Close"(reference=w272, error in=w273) -> (error out=w274:errorcluster)  [unwired: 1 in, 2 out]
              }
            }
          }
          frame "Hidden", "Hide" {
            w275 = T2."Hidden" ("State")
            n110 = property class="VI"(reference=w281, error in=w280) -> (reference out=w278:refnum<vi>, error out=w279:errorcluster, "FP.State"=w277:T2)
            n111 = Not Equal?(x=w277, y=w275) -> (x != y?=w276:bool)
            n112 = case shown="True" w276 {
              tunnel: [w286 w287] -> w282
              tunnel: w279 -> [w285 w287]
              tunnel: w278 -> [w284 _]
              tunnel: w275 -> [w283 _]
              frame True {
                n113 = invoke class="VI" method="FP.Open"(reference=w284, error in=w285, "State"=w283) -> (error out=w286:errorcluster)  [unwired: 2 in, 4 out]
              }
              frame False {
              }
            }
          }
          frame "Minimize", "Minimized" {
            w288 = T2."Minimized" ("State")
            n114 = property class="VI"(reference=w294, error in=w293) -> (reference out=w291:refnum<vi>, error out=w292:errorcluster, "FP.State"=w290:T2)
            n115 = Not Equal?(x=w290, y=w288) -> (x != y?=w289:bool)
            n116 = case shown="True" w289 {
              tunnel: [w299 w300] -> w295
              tunnel: w292 -> [w298 w300]
              tunnel: w291 -> [w297 _]
              tunnel: w288 -> [w296 _]
              frame True {
                n117 = invoke class="VI" method="FP.Open"(reference=w297, error in=w298, "State"=w296) -> (error out=w299:errorcluster)  [unwired: 2 in, 4 out]
              }
              frame False {
              }
            }
          }
          frame "Maximize", "Maximized" {
            w301 = T2."Maximized" ("State")
            n118 = property class="VI"(reference=w307, error in=w306) -> (reference out=w304:refnum<vi>, error out=w305:errorcluster, "FP.State"=w303:T2)
            n119 = Not Equal?(x=w303, y=w301) -> (x != y?=w302:bool)
            n120 = case shown="True" w302 {
              tunnel: [w312 w313] -> w308
              tunnel: w305 -> [w311 w313]
              tunnel: w304 -> [w310 _]
              tunnel: w301 -> [w309 _]
              frame True {
                n121 = invoke class="VI" method="FP.Open"(reference=w310, error in=w311, "State"=w309) -> (error out=w312:errorcluster)  [unwired: 2 in, 4 out]
              }
              frame False {
              }
            }
          }
        }
        n122 = call <vilib>:"Add State(s) to Queue__JKI_lib_State_Machine.vi"("State(s) in (\"\")"=w248) -> ("States Out"=w247:string)  [unwired: 14 in]
      }
      frame "---------- Macro ----------" {
        # "Do not put any code in this frame.\n(It is a separator no-op. You can make a copy of this frame to create a new Macro frame)"
        n123 = call <vilib>:"Add State(s) to Queue__JKI_lib_State_Machine.vi"("State(s) in (\"\")"=w318) -> ("States Out"=w317:string)  [unwired: 14 in]
      }
      frame "Macro: Initialize" {
        w320 = "Data: Initialize\nInitialize Core Data\n\nUI: Initialize\nUI: Front Panel State >> Open\n//Sim: Create Stop Event\nMacro: MQTTConnect"  # Data: Initialize Initialize Core Data  UI: Initialize UI: Front Panel State >> Open //Sim: Create Stop Event Macro: MQTTConnect
        # "Initialization Macro\n(This is called once, when the VI starts)"
        n124 = call <vilib>:"Add State(s) to Queue__JKI_lib_State_Machine.vi"("State(s) in Front (\"\")"=w320, "State(s) in (\"\")"=w324) -> ("States Out"=w323:string)  [unwired: 13 in]
      }
      frame "Macro: MQTTConnect" {
        n125 = call <vilib>:"Add State(s) to Queue__JKI_lib_State_Machine.vi"("State(s) in Front (\"\")"="MQTT: Create Client\nMQTT: Register for Events\nMQTT: Connect", "State(s) in (\"\")"=w330) -> ("States Out"=w329:string)  [unwired: 13 in]
      }
      frame "Macro: onConnection" {
        n126 = call <vilib>:"Add State(s) to Queue__JKI_lib_State_Machine.vi"("State(s) in Front (\"\")"="MQTT: Subscribe\nMQTT: PublishConnectionMessage\nMQTT: Publish State", "State(s) in (\"\")"=w336) -> ("States Out"=w335:string)  [unwired: 13 in]
      }
      frame "Macro: Change Zone" {
        n127 = Format Into String(format string="MQTT: UnregisterZone >> %s\nMQTT: RegisterZone\nMQTT: Publish Position\n", w337) -> (resulting string=w338:string)  [unwired: 2 in, 1 out]
        n128 = call <vilib>:"Add State(s) to Queue__JKI_lib_State_Machine.vi"("State(s) in Front (\"\")"=w338, "State(s) in (\"\")"=w344) -> ("States Out"=w343:string)  [unwired: 13 in]
      }
      frame "Macro: onDisconnection" {
        n129 = call <vilib>:"Add State(s) to Queue__JKI_lib_State_Machine.vi"("State(s) in (\"\")"=w349) -> ("States Out"=w348:string)  [unwired: 14 in]
      }
      frame "Macro: MQTTDisconnect" {
        n130 = call <vilib>:"Add State(s) to Queue__JKI_lib_State_Machine.vi"("State(s) in Front (\"\")"="MQTT: Unsubscribe\nMQTT: Unregister\nMQTT: PublishDisconnectionMessage\nMQTT: Disconnect\nMQTT: Destroy Client", "State(s) in (\"\")"=w355) -> ("States Out"=w354:string)  [unwired: 13 in]
      }
      frame "Macro: Exit" {
        # "Exit Macro\n(This is called once, when the VI exits)"
        n131 = Unbundle By Name(w364) -> ("Core.Close Panel on Exit?"=w363:bool)
        n132 = Select(t="UI: Front Panel State >> Close", s=w363, f="") -> (s? t:f=w360:string)
        n133 = call <vilib>:"Add State(s) to Queue__JKI_lib_State_Machine.vi"("State(s) in Front (\"\")"="//Sim: Send Stop Signal\nMacro: MQTTDisconnect", "State(s) in (\"\")"=w360, "State(s) at Back (\"\")"="Data: Cleanup\nExit") -> ("States Out"=w358:string)  [unwired: 12 in]
        n134 = call <vilib>:"Add State(s) to Queue__JKI_lib_State_Machine.vi"("State(s) in Front (\"\")"=w358, "State(s) in (\"\")"=w367) -> ("States Out"=w366:string)  [unwired: 13 in]
      }
      frame "---------- Simulation ----------" {
        # "Simulation Separator\n(You can make a copy of, or modify, this frame)"
        n135 = call <vilib>:"Add State(s) to Queue__JKI_lib_State_Machine.vi"("State(s) in (\"\")"=w372) -> ("States Out"=w371:string)  [unwired: 14 in]
      }
      frame "Sim: Create Stop Event" {
        w376 = FALSE  # stop
        n136 = Create User Event(user event datatype=w376) -> (user event=w375:refnum<user-event>)  [unwired: 1 in, 1 out]
        n137 = Bundle By Name(cluster=w374, "stop signal"=w375) -> (w373:T11)
        n138 = call <vilib>:"Add State(s) to Queue__JKI_lib_State_Machine.vi"("State(s) in (\"\")"=w380) -> ("States Out"=w379:string)  [unwired: 14 in]
      }
      frame "Sim: Destroy Stop Event" {
        n139 = Unbundle By Name(w382) -> ("stop signal"=w381:refnum<user-event>)
        n140 = Destroy User Event(user event=w381) -> ()  [unwired: 1 in, 1 out]
        n141 = call <vilib>:"Add State(s) to Queue__JKI_lib_State_Machine.vi"("State(s) in (\"\")"=w386) -> ("States Out"=w385:string)  [unwired: 14 in]
      }
      frame "Sim: Send Stop Signal" {
        n142 = Unbundle By Name(w389) -> ("stop signal"=w388:refnum<user-event>)
        n143 = Generate User Event(user event=w388, event data cluster=TRUE ("event data")) -> ()  [unwired: 2 in, 2 out]
        n144 = call <vilib>:"Add State(s) to Queue__JKI_lib_State_Machine.vi"("State(s) in (\"\")"=w393) -> ("States Out"=w392:string)  [unwired: 14 in]
      }
      frame "---------- Requests ----------" {
        # "Handling Requests\n(You can make a copy of, or modify, this frame)"
        n145 = call <vilib>:"Add State(s) to Queue__JKI_lib_State_Machine.vi"("State(s) in (\"\")"=w398) -> ("States Out"=w397:string)  [unwired: 14 in]
      }
      frame "Request: Handle Incoming" {
        n146 = Unbundle By Name(w400) -> ("project namespace"=w406:string, "Request.reply-to"=w402:string, "Client"=w408:refnum<class "Client.lvclass">, "Request.request"=w401:string)
        n147 = case shown="\"list-zones\"" w401 {
          selector: w401 -> [w414 w419 w427]
          tunnel: w400 -> [_ w422 w429]
          tunnel: [w415 w420 w428] -> w399
          frame Default {
            w416 = "Unhandled Request"  # response
            n148 = Bundle(cluster=T4 {"request"="", "reply"=variant(string "")}, "request"=w414, "reply"=w416) -> (w415:T4)
          }
          frame "list-zones" {
            n149 = Unbundle By Name(w422) -> ("TrafficMap"=w423:refnum<class "TrafficMap.lvclass">)
            n150 = call "List Zones.vi"("TrafficMap in"=w423) -> ("Zones"=w421:string[])  [unwired: 7 in, 3 out]
            n151 = Bundle(cluster=T4 {"request"="", "reply"=variant(string "")}, "request"=w419, "reply"=w421) -> (w420:T4)
          }
          frame "map" {
            n152 = Unbundle By Name(w429) -> ("TrafficMap"=w425:refnum<class "TrafficMap.lvclass">)
            n153 = call "Read Map.vi"("TrafficMap in"=w425) -> ("Map"=w424:u16[][])  [unwired: 8 in, 2 out]
            n154 = Bundle(cluster=T4 {"request"="", "reply"=variant(string "")}, "request"=w427, "reply"=w424) -> (w428:T4)
          }
        }
        n155 = Format Into String(format string="%s/%s", w406, w402) -> (resulting string=w403:string)  [unwired: 2 in, 1 out]
        n156 = call <vilib>:"Publish.vi"("error in (no error)"=w405, "Payload"=w399, "Topic Name (empty: Payload name)"=w403, "Client in"=w408) -> ("error out"=w404:errorcluster, "Client out"=w409:refnum<class "Client.lvclass">)  [unwired: 5 in, 1 out]
        n157 = Bundle By Name(cluster=w400, "Client"=w409) -> (w411:T11)
        n158 = call <vilib>:"Add State(s) to Queue__JKI_lib_State_Machine.vi"("State(s) in (\"\")"=w413) -> ("States Out"=w412:string)  [unwired: 14 in]
      }
      frame "---------- MQTT ----------" {
        # "MQTT Separator\n(You can make a copy of, or modify, this frame)"
        n159 = call <vilib>:"Add State(s) to Queue__JKI_lib_State_Machine.vi"("State(s) in (\"\")"=w434) -> ("States Out"=w433:string)  [unwired: 14 in]
      }
      frame "MQTT: Create Client" {
        # "Set JKI-JSON as the Serializer Class"
        n160 = call <vilib>:"Create MQTT Client.vi"("error in (no error)"=w441) -> ("error out"=w436:errorcluster, "Client out"=w439:refnum<class "Client.lvclass">)  [unwired: 9 in]
        n161 = call <vilib>:"Set Serializer.vi"("error in (no error)"=w436, "Serializer (default: Flattened String)"=refnum<class "Serializer.JKI-JSON.lvclass"> refnum ("Serializer.JKI-JSON.lvclass"), "MQTT_Base"=w439) -> ("error out"=w435:errorcluster, "MQTT_Base out"=w438:refnum<class "Client.lvclass">)  [unwired: 7 in]
        n162 = Bundle By Name(cluster=w443, "Client"=w438) -> (w442:T11)
        n163 = call <vilib>:"Add State(s) to Queue__JKI_lib_State_Machine.vi"("State(s) in (\"\")"=w445) -> ("States Out"=w444:string)  [unwired: 14 in]
      }
      frame "MQTT: Register for Events" {
        n164 = Unbundle By Name(w454) -> ("Client"=w452:refnum<class "Client.lvclass">, "stop signal"=w446:refnum<user-event>)
        n165 = call <vilib>:"Read Public Events.vi"("error in (no error)"=w450, "Client in"=w452) -> ("error out"=w448:errorcluster, "Client Public Events"=w453:T14, "Client out"=w451:refnum<class "Client.lvclass">)  [unwired: 7 in]
        n166 = register-events(error in=w448, w453, w446) -> (reference out=w449:refnum<event-registration>, error out=w447:errorcluster)  [unwired: 1 in]
        n167 = Bundle By Name(cluster=w454, "Client"=w451) -> (w455:T11)
        n168 = call <vilib>:"Add State(s) to Queue__JKI_lib_State_Machine.vi"("State(s) in (\"\")"=w457) -> ("States Out"=w456:string)  [unwired: 14 in]
      }
      frame "MQTT: Connect" {
        n169 = Unbundle By Name(w478) -> ("server address"=w471:string, "Client"=w474:refnum<class "Client.lvclass">, "project namespace"=w463:string, "Client Name"=w462:string)
        n170 = call <vilib>:"Start.vi"("error in (no error)"=w473, "MQTT_Base in"=w474) -> ("error out"=w476:errorcluster, "MQTT_Base out"=w475:refnum<class "Client.lvclass">)  [unwired: 7 in, 1 out]
        n171 = call <vilib>:"Flatten To JSON String.vi"("Variant"=cluster{"message":string} {"message"="unexpected disconnection"}) -> ("JSON String"=w458:string)  [unwired: 9 in, 1 out]
        n172 = Format Into String(format string="%s/%s/will", w463, w462) -> (resulting string=w464:string)  [unwired: 2 in, 1 out]
        n173 = Bundle By Name(cluster=T5 {"Reserved"=FALSE, "Clean Session"=FALSE, "Will Flag"=FALSE, "Will QoS 1"=FALSE, "Will QoS 2"=FALSE, "Will Retain"=FALSE, "Password Flag"=FALSE, "User Name Flag"=FALSE} ("Connect Flags"), "Will Flag"=TRUE) -> (w466:T5)
        n174 = Bundle By Name(cluster=T6 {"Will Topic"="", "Will Message"="", "Username"="", "Password"=""} ("Payload"), "Will Topic"=w464, "Will Message"=w458) -> (w460:T6)
        n175 = call <vilib>:"Connect to Server.vi"("Connect Flags"=w466, "Keep Alive (s)"=u16 3600, "Payload"=w460, "error in (no error)"=w476, "address (localhost)"=w471, "Client in"=w475) -> ("error out"=w472:errorcluster, "Client out"=w470:refnum<class "Client.lvclass">)  [unwired: 2 in, 2 out]
        n176 = Bundle By Name(cluster=w478, "Client"=w470) -> (w479:T11)
        n177 = call <vilib>:"Add State(s) to Queue__JKI_lib_State_Machine.vi"("State(s) in (\"\")"=w481) -> ("States Out"=w480:string)  [unwired: 14 in]
      }
      frame "MQTT: Subscribe" {
        n178 = Unbundle By Name(w491) -> ("project namespace"=w488:string, "Client Name"=w487:string, "Client"=w486:refnum<class "Client.lvclass">)
        n179 = Format Into String(format string="%s/users/%s/#", w488, w487) -> (resulting string=w482:string)  [unwired: 2 in, 1 out]
        n180 = call <vilib>:"Subscribe (SingleTopic).vi"("error in (no error)"=w484, "Topic Filter"=w482, "MQTT_Base in"=w486) -> ("error out"=w483:errorcluster, "MQTT_Base out"=w485:refnum<class "Client.lvclass">)  [unwired: 7 in]
        n181 = Bundle By Name(cluster=w491, "Client"=w485) -> (w492:T11)
        n182 = call <vilib>:"Add State(s) to Queue__JKI_lib_State_Machine.vi"("State(s) in (\"\")"=w494) -> ("States Out"=w493:string)  [unwired: 14 in]
      }
      frame "MQTT: Unsubscribe" {
        n183 = Unbundle By Name(w504) -> ("project namespace"=w497:string, "Client Name"=w495:string, "Client"=w502:refnum<class "Client.lvclass">)
        n184 = Format Into String(format string="%s/users/%s/#", w497, w495) -> (resulting string=w496:string)  [unwired: 2 in, 1 out]
        n185 = call <vilib>:"Unsubscribe (SingleTopic).vi"("error in (no error)"=w500, "Topic Filter"=w496, "MQTT_Base in"=w502) -> ("error out"=w499:errorcluster, "MQTT_Base out"=w501:refnum<class "Client.lvclass">)  [unwired: 7 in]
        n186 = Bundle By Name(cluster=w504, "Client"=w501) -> (w505:T11)
        n187 = call <vilib>:"Add State(s) to Queue__JKI_lib_State_Machine.vi"("State(s) in (\"\")"=w507) -> ("States Out"=w506:string)  [unwired: 14 in]
      }
      frame "MQTT: UnregisterZone" {
        n188 = Unbundle By Name(w510) -> ("project namespace"=w511:string, "Client"=w515:refnum<class "Client.lvclass">)  [unwired: 1 out]
        n189 = Empty String/Path?(string/path=w509) -> (empty?=w508:bool)
        n190 = case shown="False" w508 {
          tunnel: w515 -> [w528 w530]
          tunnel: [w527 w530] -> w514
          tunnel: w513 -> [w526 w529]
          tunnel: [w525 w529] -> w512
          tunnel: w511 -> [w523 _]
          tunnel: w509 -> [w520 _]
          frame False {
            n191 = Format Into String(format string="%s/traffic-data/zone/%s/#", w523, w520) -> (resulting string=w522:string)  [unwired: 2 in, 1 out]
            n192 = Wait (ms)(milliseconds to wait=u32 200) -> ()  [unwired: 1 out]
            n193 = call <vilib>:"Unsubscribe (SingleTopic).vi"("error in (no error)"=w526, "Topic Filter"=w522, "MQTT_Base in"=w528) -> ("error out"=w525:errorcluster, "MQTT_Base out"=w527:refnum<class "Client.lvclass">)  [unwired: 7 in]
          }
          frame True {
          }
        }
        n194 = Bundle By Name(cluster=w510, "Client"=w514) -> (w517:T11)
        n195 = call <vilib>:"Add State(s) to Queue__JKI_lib_State_Machine.vi"("State(s) in (\"\")"=w519) -> ("States Out"=w518:string)  [unwired: 14 in]
      }
      frame "MQTT: RegisterZone" {
        n196 = Unbundle By Name(w538) -> ("project namespace"=w540:string, "Client"=w536:refnum<class "Client.lvclass">)  [unwired: 1 out]
        n197 = Unbundle By Name(w538) -> ("TrafficMap"=w539:refnum<class "TrafficMap.lvclass">)
        n198 = call "Read Position.vi"("TrafficMap in"=w539) -> ("Position"=w537:string)  [unwired: 8 in, 2 out]
        n199 = Format Into String(format string="%s/traffic-data/zone/%s/#", w540, w537) -> (resulting string=w532:string)  [unwired: 2 in, 1 out]
        "Zone registered" <- w532
        n200 = call <vilib>:"Subscribe (SingleTopic).vi"("error in (no error)"=w535, "Topic Filter"=w532, "MQTT_Base in"=w536) -> ("error out"=w534:errorcluster, "MQTT_Base out"=w533:refnum<class "Client.lvclass">)  [unwired: 7 in]
        n201 = Wait (ms)(milliseconds to wait=u32 200) -> ()  [unwired: 1 out]
        n202 = Bundle By Name(cluster=w538, "Client"=w533) -> (w543:T11)
        n203 = call <vilib>:"Add State(s) to Queue__JKI_lib_State_Machine.vi"("State(s) in (\"\")"=w545) -> ("States Out"=w544:string)  [unwired: 14 in]
      }
      frame "MQTT: Publish State" {
        n204 = Unbundle By Name(w557) -> ("project namespace"=w552:string, "Client Name"=w551:string, "Client"=w554:refnum<class "Client.lvclass">)
        n205 = Format Into String("car state") -> (resulting string=w546:string)  [unwired: 3 in, 1 out]
        n206 = Format Into String(format string="%s/users/%s/state", w552, w551) -> (resulting string=w550:string)  [unwired: 2 in, 1 out]
        n207 = call <vilib>:"Publish.vi"("error in (no error)"=w549, "Payload"=w546, "Topic Name (empty: Payload name)"=w550, "Client in"=w554) -> ("error out"=w548:errorcluster, "Client out"=w555:refnum<class "Client.lvclass">)  [unwired: 5 in, 1 out]
        n208 = Bundle By Name(cluster=w557, "Client"=w555) -> (w558:T11)
        n209 = call <vilib>:"Add State(s) to Queue__JKI_lib_State_Machine.vi"("State(s) in (\"\")"=w560) -> ("States Out"=w559:string)  [unwired: 14 in]
      }
      frame "MQTT: Publish Position" {
        n210 = Unbundle By Name(w572) -> ("project namespace"=w567:string, "Client Name"=w566:string, "Client"=w569:refnum<class "Client.lvclass">, "TrafficMap"=w562:refnum<class "TrafficMap.lvclass">)
        n211 = call "Read Position.vi"("TrafficMap in"=w562) -> ("Position"=w561:string)  [unwired: 8 in, 2 out]
        n212 = Format Into String(format string="%s/users/%s/position", w567, w566) -> (resulting string=w565:string)  [unwired: 2 in, 1 out]
        n213 = call <vilib>:"Publish.vi"("error in (no error)"=w564, "Payload"=w561, "Topic Name (empty: Payload name)"=w565, "Client in"=w569) -> ("error out"=w563:errorcluster, "Client out"=w570:refnum<class "Client.lvclass">)  [unwired: 5 in, 1 out]
        n214 = Bundle By Name(cluster=w572, "Client"=w570) -> (w573:T11)
        n215 = call <vilib>:"Add State(s) to Queue__JKI_lib_State_Machine.vi"("State(s) in (\"\")"=w575) -> ("States Out"=w574:string)  [unwired: 14 in]
      }
      frame "MQTT: RequestZoneList" {
        n216 = Unbundle By Name(w590) -> ("project namespace"=w578:string, "Client Name"=w577:string, "Client"=w587:refnum<class "Client.lvclass">)  [unwired: 1 out]
        n217 = Format Into String(format string="%s/users/%s/inbox", w578, w577) -> (resulting string=w580:string)  [unwired: 2 in, 1 out]
        n218 = Format Into String(format string="%s/traffic-data/request", w578) -> (resulting string=w585:string)  [unwired: 2 in, 1 out]
        n219 = Bundle By Name(cluster=T7 {"request"="", "reply-to"=""} ("Request Payload"), "request"="list-zones" ("Request"), "reply-to"=w580) -> (w582:T7)
        n220 = call <vilib>:"Publish.vi"("error in (no error)"=w584, "Payload"=w582, "Topic Name (empty: Payload name)"=w585, "Client in"=w587) -> ("error out"=w583:errorcluster, "Client out"=w588:refnum<class "Client.lvclass">)  [unwired: 5 in, 1 out]
        n221 = Bundle By Name(cluster=w590, "Client"=w588) -> (w591:T11)
        n222 = call <vilib>:"Add State(s) to Queue__JKI_lib_State_Machine.vi"("State(s) in (\"\")"=w593) -> ("States Out"=w592:string)  [unwired: 14 in]
      }
      frame "MQTT: RequestTrafficMap" {
        n223 = Unbundle By Name(w608) -> ("project namespace"=w596:string, "Client Name"=w595:string, "Client"=w605:refnum<class "Client.lvclass">)  [unwired: 1 out]
        n224 = Format Into String(format string="%s/users/%s/inbox", w596, w595) -> (resulting string=w598:string)  [unwired: 2 in, 1 out]
        n225 = Format Into String(format string="%s/traffic-data/request", w596) -> (resulting string=w603:string)  [unwired: 2 in, 1 out]
        n226 = Bundle By Name(cluster=T7 {"request"="", "reply-to"=""} ("Request Payload"), "request"="map" ("Request"), "reply-to"=w598) -> (w600:T7)
        n227 = call <vilib>:"Publish.vi"("error in (no error)"=w602, "Payload"=w600, "Topic Name (empty: Payload name)"=w603, "Client in"=w605) -> ("error out"=w601:errorcluster, "Client out"=w606:refnum<class "Client.lvclass">)  [unwired: 5 in, 1 out]
        n228 = Bundle By Name(cluster=w608, "Client"=w606) -> (w609:T11)
        n229 = call <vilib>:"Add State(s) to Queue__JKI_lib_State_Machine.vi"("State(s) in (\"\")"=w611) -> ("States Out"=w610:string)  [unwired: 14 in]
      }
      frame "MQTT: PublishConnectionMessage" {
        n230 = Unbundle By Name(w625) -> ("project namespace"=w620:string, "Client Name"=w619:string, "Client"=w622:refnum<class "Client.lvclass">, "Node type"=w615:T10)
        n231 = Format Into String(w615) -> (resulting string=w614:string)  [unwired: 3 in, 1 out]
        n232 = Format Into String(format string="%s/users/%s/connect", w620, w619) -> (resulting string=w618:string)  [unwired: 2 in, 1 out]
        n233 = Bundle(cluster=T8 {"Node type"=""} ("Connect payload"), "Node type"=w614) -> (w613:T8)
        n234 = call <vilib>:"Publish.vi"("error in (no error)"=w617, "Payload"=w613, "Topic Name (empty: Payload name)"=w618, "Client in"=w622) -> ("error out"=w616:errorcluster, "Client out"=w623:refnum<class "Client.lvclass">)  [unwired: 5 in, 1 out]
        n235 = Bundle By Name(cluster=w625, "Client"=w623) -> (w626:T11)
        n236 = call <vilib>:"Add State(s) to Queue__JKI_lib_State_Machine.vi"("State(s) in (\"\")"=w628) -> ("States Out"=w627:string)  [unwired: 14 in]
      }
      frame "MQTT: PublishDisconnectionMessage" {
        n237 = Unbundle By Name(w641) -> ("project namespace"=w636:string, "Client Name"=w635:string, "Client"=w638:refnum<class "Client.lvclass">)
        n238 = Format Into String(format string="%s/users/%s/disconnect", w636, w635) -> (resulting string=w634:string)  [unwired: 2 in, 1 out]
        n239 = call "Formatted Timestamp.vi"() -> ("String Formatted timestamp"=w630:string)  [unwired: 11 in]
        n240 = Bundle(cluster=T9 {"timestamp"=""} ("Disconnect payload"), "timestamp"=w630) -> (w629:T9)
        n241 = call <vilib>:"Publish.vi"("error in (no error)"=w633, "Payload"=w629, "Topic Name (empty: Payload name)"=w634, "Client in"=w638) -> ("error out"=w632:errorcluster, "Client out"=w639:refnum<class "Client.lvclass">)  [unwired: 5 in, 1 out]
        n242 = Bundle By Name(cluster=w641, "Client"=w639) -> (w642:T11)
        n243 = call <vilib>:"Add State(s) to Queue__JKI_lib_State_Machine.vi"("State(s) in (\"\")"=w644) -> ("States Out"=w643:string)  [unwired: 14 in]
      }
      frame "MQTT: Handle App Message" {
        n244 = Unbundle By Name(w651) -> ("Client Name"=w645:string, "Client"=w658:refnum<class "Client.lvclass">, "AppMessage"=w648:refnum<class "PUBLISH.lvclass">)
        n245 = call <vilib>:"Read Payload.vi"("ControlPacket in"=w648) -> ("Payload"=w647:u8[])  [unwired: 9 in, 1 out]
        n246 = call <vilib>:"getTopicName.vi"("PUBLISH in"=w648) -> ("Topic"=w657:string, "PUBLISH out"=w659:refnum<class "PUBLISH.lvclass">)  [unwired: 8 in, 1 out]
        "Topic" <- w657
        n247 = property on="Car Client Status" class="MCListbox (strict)"() -> ("ItemNames"=w655:string[][])  [unwired: 2 in, 2 out]
        n248 = Byte Array To String(unsigned byte array=w647) -> (string=→"Raw Packet String":string)
        n249 = call "topic_to_Array.vi"("Topic"=w657) -> ("Topic (Array)"=w661:string[])  [unwired: 10 in]
        n250 = Delete From Array(array=w661) -> (deleted portion=w660:string, array with subset deleted=w656:string[])  [unwired: 2 in]
        n251 = case shown="\"inbox\"" w660 {
          tunnel: w659 -> [w669 w674 w685 w723 w743 w757 w782 w799]
          tunnel: w658 -> [w670 w675 w688 w722 w742 w756 w781 _]
          tunnel: w656 -> [_ _ _ w721 _ w755 w780 w806]
          tunnel: w655 -> [w667 w678 w687 w711 w739 w745 w772 w797]
          tunnel: [w667 w678 w687 w717 w739 w751 w775 w801] -> w653
          tunnel: w651 -> [w666 w677 w680 w714 w741 w748 w771 w796]
          tunnel: [w666 w676 w681 w714 w741 w748 w771 w796] -> w650
          tunnel: [_ "Request: Handle Incoming" w679 _ _ _ _ _] -> w649
          tunnel: w645 -> [_ _ _ _ _ _ _ _]
          frame Default {
            n252 = call "Decode Publish Packet.vim"("PUBLISH"=w669, "Client in"=w670) -> ("Payload"=→"Payload":variant)  [unwired: 6 in, 3 out]
          }
          frame "request" {
            n253 = call "Decode Publish Packet.vim"("Payload type"=T7 {"request"="", "reply-to"=""} ("Request Payload"), "PUBLISH"=w674, "Client in"=w675) -> ("Payload"=w672:T7)  [unwired: 5 in, 3 out]
            n254 = Bundle By Name(cluster=w677, "Request"=w672) -> (w676:T11)
          }
          frame "inbox" {
            n255 = call "Decode Publish Packet.vim"("Payload type"=T4 {"request"="", "reply"=variant} ("Response Payload"), "PUBLISH"=w685, "Client in"=w688) -> ("Payload"=w684:T4)  [unwired: 5 in, 3 out]
            n256 = Unbundle(w684) -> ("request"=w683:string, "reply"=w682:variant)
            n257 = case shown="\"list-zones\"" w683 {
              tunnel: w682 -> [_ w699 w709]
              tunnel: [w689 w693 w706] -> w681
              tunnel: w680 -> [w689 w691 w704]
              tunnel: [_ "UI: Update Zone List" "UI: Update Zone Map"] -> w679
              frame "False", Default {
              }
              frame "list-zones" {
                w696 = string[] []
                n258 = Unbundle By Name(w691) -> ("TrafficMap"=w690:refnum<class "TrafficMap.lvclass">)
                n259 = call <vilib>:"Adapt To Type.vi"("Type and Defaults"=w696, "Variant in"=w699) -> ("error out"=w698:errorcluster, "Variant out"=w697:variant)  [unwired: 8 in]
                n260 = Variant To Data(error in=w698, type=w696, Variant=w697) -> (data=w694:string[])  [unwired: 1 out]
                n261 = call "Create TrafficMap.vi"("TrafficMap in"=w690, "Zones"=w694) -> ("TrafficMap"=w695:refnum<class "TrafficMap.lvclass">)  [unwired: 8 in, 1 out]
                n262 = Bundle By Name(cluster=w691, "TrafficMap"=w695) -> (w693:T11)
              }
              frame "map" {
                w703 = u16[][] []  # Map
                n263 = Unbundle By Name(w704) -> ("TrafficMap"=w702:refnum<class "TrafficMap.lvclass">)
                n264 = call <vilib>:"Adapt To Type.vi"("Type and Defaults"=w703, "Variant in"=w709) -> ("error out"=w708:errorcluster, "Variant out"=w707:variant)  [unwired: 8 in]
                n265 = Variant To Data(error in=w708, type=w703, Variant=w707) -> (data=w701:u16[][])  [unwired: 1 out]
                n266 = call "Write Map.vi"("Map"=w701, "TrafficMap in"=w702) -> ("TrafficMap out"=w700:refnum<class "TrafficMap.lvclass">)  [unwired: 8 in, 1 out]
                n267 = Bundle By Name(cluster=w704, "TrafficMap"=w700) -> (w706:T11)
              }
            }
          }
          frame "state" {
            n268 = Delete From Array(array=w721) -> (deleted portion=w718:string)  [unwired: 2 in, 1 out]
            n269 = Index Array(array=w711, index (col)=0 ("disabled index (col)")) -> (element=w719:string[])  [unwired: 1 in]
            n270 = call "Decode Publish Packet.vim"("Payload type"="", "PUBLISH"=w723, "Client in"=w722) -> ("Payload"=w715:string)  [unwired: 5 in, 3 out]
            n271 = Search 1D Array(1D array=w719, element=w718) -> (index of element=w713:i32)  [unwired: 1 in]
            n272 = Index Array(array=w711, index (row)=w713, index (col)=2) -> (element=w710:string)
            n273 = case shown="-1" w713 {
              selector: w713 -> [_ w731]
              tunnel: [w728 w733] -> w717
              tunnel: w711 -> [w727 w734]
              tunnel: w715 -> [w726 w736]
              tunnel: w718 -> [w725 w735]
              tunnel: w710 -> [w724 w730]
              frame -1 {
                n274 = Build Array(w725, w726, w724) -> (w729:string[])
                n275 = Build Array (concatenate)(w729, w727) -> (w728:string[][])
              }
              frame Default {
                n276 = Build Array(w735, w736, w730) -> (w732:string[])
                n277 = Replace Array Subset(array=w734, new element=w732, index (row)=w731) -> (w733:string[][])  [unwired: 1 in]
              }
            }
          }
          frame "nb-cars" {
            n278 = call "Decode Publish Packet.vim"("Payload type"=u32 0 ("index (col)"), "PUBLISH"=w743, "Client in"=w742) -> ("Payload"=→"Nb Cars in Current Zone":u32, "Topic"=→"Incoming topic":string)  [unwired: 5 in, 2 out]
          }
          frame "position" {
            n279 = Delete From Array(array=w755) -> (deleted portion=w752:string)  [unwired: 2 in, 1 out]
            n280 = Index Array(array=w745, index (col)=0 ("disabled index (col)")) -> (element=w753:string[])  [unwired: 1 in]
            n281 = call "Decode Publish Packet.vim"("Payload type"="", "PUBLISH"=w757, "Client in"=w756) -> ("Payload"=w749:string)  [unwired: 5 in, 3 out]
            n282 = Search 1D Array(1D array=w753, element=w752) -> (index of element=w747:i32)  [unwired: 1 in]
            n283 = Index Array(array=w745, index (row)=w747, index (col)=1) -> (element=w744:string)
            n284 = case shown="Default" w747 {
              selector: w747 -> [_ w766]
              tunnel: [w762 w768] -> w751
              tunnel: w745 -> [w761 w769]
              tunnel: w749 -> [w759 w764]
              tunnel: w752 -> [w760 w770]
              tunnel: w744 -> [w758 w765]
              frame -1 {
                n285 = Build Array(w760, w758, w759) -> (w763:string[])
                n286 = Build Array (concatenate)(w763, w761) -> (w762:string[][])
              }
              frame Default {
                n287 = Build Array(w770, w765, w764) -> (w767:string[])
                n288 = Replace Array Subset(array=w769, new element=w767, index (row)=w766) -> (w768:string[][])  [unwired: 1 in]
              }
            }
          }
          frame "disconnect" {
            n289 = Delete From Array(array=w780) -> (deleted portion=w777:string)  [unwired: 2 in, 1 out]
            n290 = Index Array(array=w772, index (col)=0 ("disabled index (col)")) -> (element=w778:string[])  [unwired: 1 in]
            n291 = call "Decode Publish Packet.vim"("Payload type"="", "PUBLISH"=w782, "Client in"=w781) -> ("Payload"=w773:string)  [unwired: 5 in, 3 out]
            n292 = Search 1D Array(1D array=w778, element=w777) -> (index of element=w776:i32)  [unwired: 1 in]
            n293 = case shown="Default" w776 {
              selector: w776 -> [_ w793]
              tunnel: [w787 w795] -> w775
              tunnel: w772 -> [w786 w794]
              tunnel: w773 -> [w783 w789]
              tunnel: w777 -> [w785 _]
              frame -1 {
                n294 = Build Array(w785, "" ("element"), w783) -> (w788:string[])
                n295 = Build Array (concatenate)(w788, w786) -> (w787:string[][])
              }
              frame Default {
                n296 = Index Array(array=w794, index (row)=w793) -> (element=w792:string[])  [unwired: 1 in]
                n297 = Replace Array Subset(array=w792, new element=w789, index=2) -> (w790:string[])
                n298 = Replace Array Subset(array=w794, new element=w790, index (row)=w793) -> (w795:string[][])  [unwired: 1 in]
              }
            }
          }
          frame "will" {
            n299 = Delete From Array(array=w806) -> (deleted portion=w803:string)  [unwired: 2 in, 1 out]
            n300 = Index Array(array=w797, index (col)=0 ("disabled index (col)")) -> (element=w804:string[])  [unwired: 1 in]
            n301 = call <vilib>:"Read Payload.vi"("ControlPacket in"=w799) -> ("Payload"=w800:u8[])  [unwired: 9 in, 1 out]
            n302 = Search 1D Array(1D array=w804, element=w803) -> (index of element=w802:i32)  [unwired: 1 in]
            n303 = Byte Array To String(unsigned byte array=w800) -> (string=w798:string)
            n304 = case shown="Default" w802 {
              selector: w802 -> [_ w815]
              tunnel: [w811 w817] -> w801
              tunnel: w797 -> [w810 w818]
              tunnel: w798 -> [w807 w814]
              tunnel: w803 -> [w809 w819]
              frame -1 {
                n305 = Build Array(w809, "" ("element"), w807) -> (w812:string[])
                n306 = Build Array (concatenate)(w812, w810) -> (w811:string[][])
              }
              frame Default {
                n307 = Build Array(w819, "" ("element"), w814) -> (w816:string[])
                n308 = Replace Array Subset(array=w818, new element=w816, index (row)=w815) -> (w817:string[][])  [unwired: 1 in]
              }
            }
          }
        }
        n309 = Array Subset(array=w653, length (row)=50 ("length")) -> (w652:string[][])  [unwired: 3 in]
        n310 = property on="Car Client Status" class="MCListbox (strict)"("ItemNames"=w652) -> ()  [unwired: 2 in, 2 out]
        n311 = call <vilib>:"Add State(s) to Queue__JKI_lib_State_Machine.vi"("State(s) in Front (\"\")"=w649, "State(s) in (\"\")"=w665) -> ("States Out"=w664:string)  [unwired: 13 in]
      }
      frame "MQTT: Disconnect" {
        n312 = Unbundle By Name(w827) -> ("Client"=w825:refnum<class "Client.lvclass">)
        n313 = call <vilib>:"Disconnect from Server.vi"("error in (no error)"=w820, "Client in"=w825) -> ("error out"=w821:errorcluster, "Client out"=w824:refnum<class "Client.lvclass">)  [unwired: 7 in, 1 out]
        n314 = call <vilib>:"Stop.vi"("error in (no error)"=w821, "MQTT_Base in"=w824) -> ("error out"=w822:errorcluster, "MQTT_Base out"=w823:refnum<class "Client.lvclass">)  [unwired: 7 in, 1 out]
        n315 = Bundle By Name(cluster=w827, "Client"=w823) -> (w828:T11)
        n316 = call <vilib>:"Add State(s) to Queue__JKI_lib_State_Machine.vi"("State(s) in (\"\")"=w830) -> ("States Out"=w829:string)  [unwired: 14 in]
      }
      frame "MQTT: Unregister" {
        n317 = Unregister For Events(event registration refnum=w834, error in=w833) -> (error out=w832:errorcluster)
        n318 = call <vilib>:"Add State(s) to Queue__JKI_lib_State_Machine.vi"("State(s) in (\"\")"=w836) -> ("States Out"=w835:string)  [unwired: 14 in]
      }
      frame "MQTT: Destroy Client" {
        n319 = Unbundle By Name(w841) -> ("Client"=w840:refnum<class "Client.lvclass">)
        n320 = call-dynamic "Destroy.vi"("error in (no error)"=w839, "MQTT_Base in"=w840) -> ("error out"=w838:errorcluster)  [unwired: 8 in, 1 out]
        n321 = call <vilib>:"Add State(s) to Queue__JKI_lib_State_Machine.vi"("State(s) in (\"\")"=w843) -> ("States Out"=w842:string)  [unwired: 14 in]
      }
    }
  }
